vi "wrap.GetType.vi"(0 "class.GLue in":refnum<class "class.GLue.lvclass">, 11 "error in (no error)":errorcluster, 13 "Index":i32=-1) -> (4 "class.GLue out":refnum<class "class.GLue.lvclass">, 8 "Type":T1, 15 "error out":errorcluster)   [LabVIEW 2014, in "GLue.lvlib" / "class.GLue.lvclass"]
uses:
  class.GLue.lvclass
  typedef.Types.ctl
  class.GLue.lvclass/class.GLue.ctl
  Resources/GLue.dll
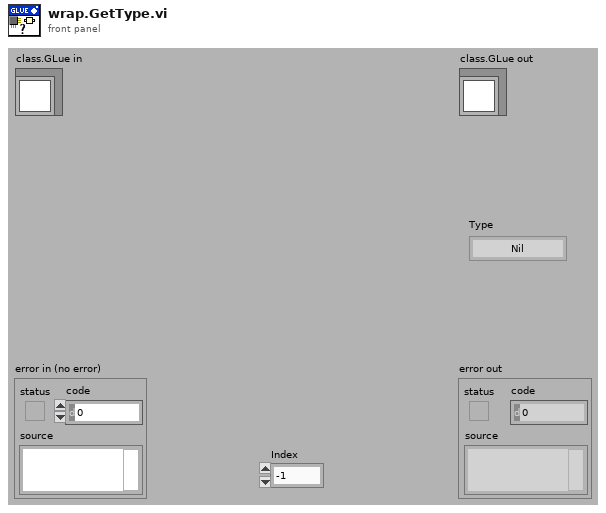
[diagram p1: front panel]
types:
  T1 = typedef "GLue.lvlib/class.GLue.lvclass/typedef.Types.ctl" = enum16{"Nil", "Bool", "LightUserData", "Number", "String", "Table", "Function", "UserData", "Thread"}
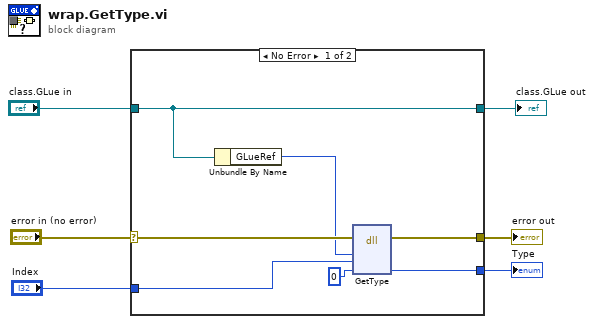
[diagram p0: block diagram]
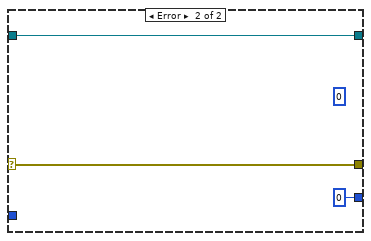
[diagram p2: hidden frame]
diagram:
  n1 = case shown="No Error" "error in (no error)" {
    selector: "error in (no error)" -> [w12 w16]
    tunnel: [w11 w16] -> w5
    tunnel: [w13 w15] -> w3
    tunnel: "class.GLue in" -> [w13 w15]
    tunnel: [w8 0 ("TopType")] -> w2
    tunnel: "Index" -> [w7 _]
    frame No Error {
      n2 = Unbundle By Name(w13) -> ("GLueRef"=w10:i64)
      n3 = dll-call lib="C:/Users/Antonie/Documents/work/glue/trunk/Resources/GLue.dll" fn="GetType"(error in=w12, "GLue"=w10, "Index"=w7, "Type"=0 ("Bool")) -> (error out=w11:errorcluster, "Type"=w8:i32)  [unwired: 5 in, 1 out]
    }
    frame Error {
      (unwired) 0 ("Size")
    }
  }
  "error out" <- w5
  "class.GLue out" <- w3
  "Type" <- w2
